vi "rotate_boat_overlays.vi"(8 "Overlay References In":T3, 9 "Rudder Setpoint":T1 min=-0.95 max=0.95 scale=1.0..-1.0, 10 "Sail Setpoints":T2 {"MainSailSuggestion" min=0.0 max=1.0; "JibSailSuggestion" min=0.0 max=1.0}, 11 "Heading":dbl) -> (1 "Rotated Boat Icon Bitmap Out":u32[][](array[colorbox]), 3 "Boat Icon Out":T4(plugin-control))   [LabVIEW 2013]
doc: "Rotates icon images of the boat and sails and overlays them on each other to create a representation of the current state of the robot. Also converts the output image to a bitmap for easy overlay on the mission map.\n\norigininally by Jason Curtis\nAdapted 4/5/2014 by Mac-I Crowell"
uses:
  TypeDef/boat_overlay_references.ctl
  <vilib>/vision/Image Controls.llb/IMAQ Image.ctl
  cRIO_Code/Data/TypeDefs/Sail Set Suggestions.ctl
  cRIO_Code/Data/TypeDefs/Rudder Set Suggestions.ctl
  <vilib>/vision/NI_Vision_Development_Module.lvlib
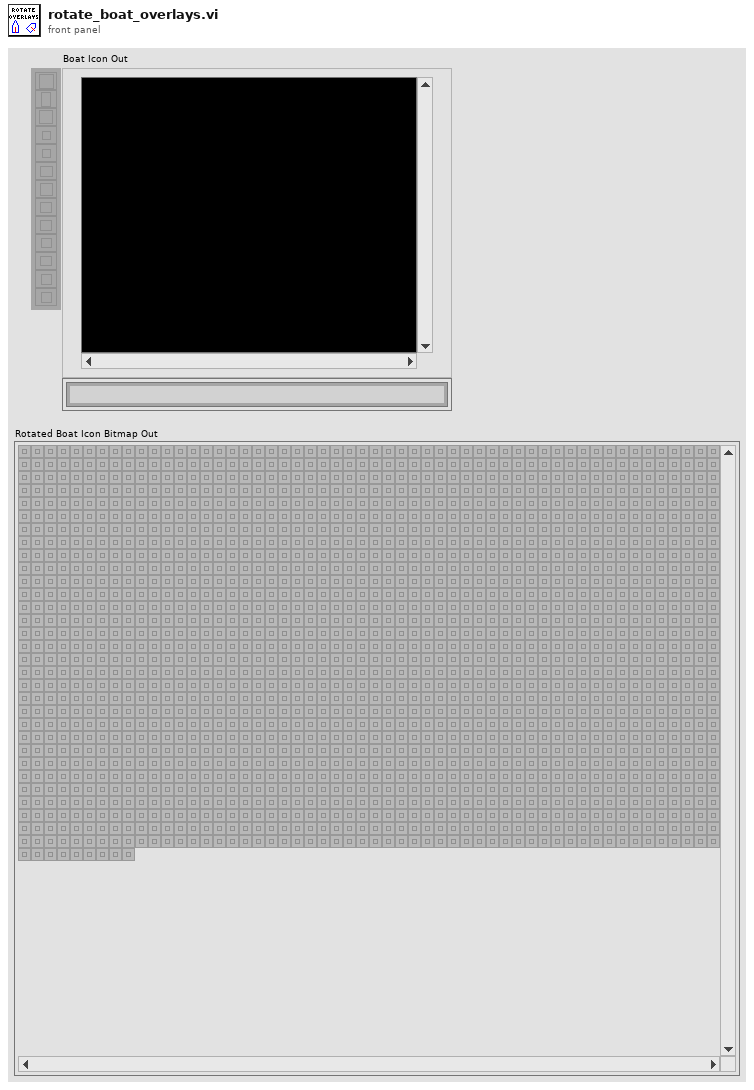
[diagram p1: front panel]
types:
  T1 = typedef "Rudder Set Suggestions.ctl" = dbl
  T2 = typedef "Sail Set Suggestions.ctl" = cluster{"MainSailSuggestion":dbl, "JibSailSuggestion":dbl}
  T3 = typedef "boat_overlay_references.ctl" = cluster{"Boat Icon, Unrotated":T4, "Boat Icon, Rotated":T4, "Mainsail Icon, Unrotated":T4, "Mainsail Icon, Rotated":T4, "Jib Icon, Rotated":T4, "Jib Icon, Unrotated":T4, "Rudder Icon, Rotated":T4, "Rudder Icon, Unrotated":T4}
  T4 = typedef "IMAQ Image.ctl" = refnum<image>
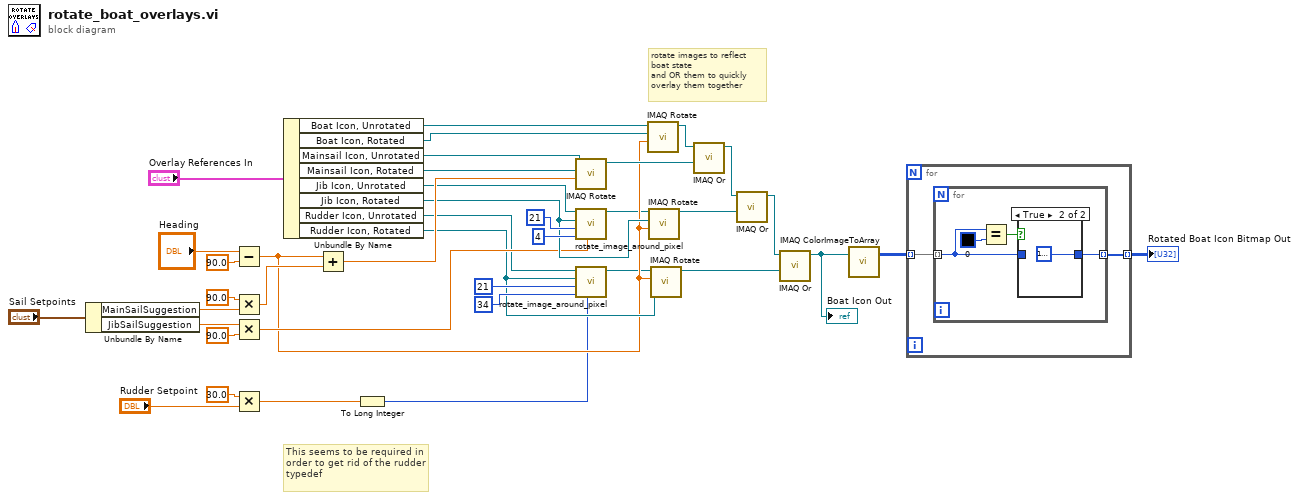
[diagram p0: block diagram]
diagram:
  # "This seems to be required in order to get rid of the rudder typedef"
  # "rotate images to reflect\nboat state\nand OR them to quickly \noverlay them together"
  n1 = Unbundle By Name("Sail Setpoints") -> ("MainSailSuggestion"=w24:dbl, "JibSailSuggestion"=w21:dbl)
  n2 = Subtract(x="Heading", y=90.0) -> (x-y=w8:dbl)
  n3 = Multiply(x=90.0 ("y"), y=w24) -> (x*y=w29:dbl)
  n4 = Multiply(x=w21, y=90.0) -> (x*y=w10:dbl)
  n5 = Multiply(x=30.0 ("y"), y="Rudder Setpoint") -> (x*y=w16:T1)
  n6 = Unbundle By Name("Overlay References In") -> ("Boat Icon, Unrotated"=w39:T4, "Boat Icon, Rotated"=w38:T4, "Mainsail Icon, Unrotated"=w36:T4, "Mainsail Icon, Rotated"=w37:T4, "Jib Icon, Unrotated"=w3:T4, "Jib Icon, Rotated"=w11:T4, "Rudder Icon, Unrotated"=w6:T4, "Rudder Icon, Rotated"=w9:T4)
  n7 = Add(x=w8, y=w29) -> (x+y=w30:dbl)
  n8 = To Long Integer(number=w16) -> (32bit integer=w7:i32)
  n9 = call "IMAQ Rotate"("Angle (degrees)"=w30, "Image Dst"=w37, "Image Src"=w36) -> ("Image Dst Out"=w34:T4)  [unwired: 7 in, 1 out]
  n10 = call "rotate_image_around_pixel.vi"("Angle (degrees)"=w10, "Y Pixel"=4, "X Pixel"=21, "Image Dst"=w11, "Image Src"=w3) -> ("Image Dst Out"=w2:T4)  [unwired: 6 in]
  n11 = call "rotate_image_around_pixel.vi"("Angle (degrees)"=w7, "Y Pixel"=34, "X Pixel"=21, "Image Dst"=w9, "Image Src"=w6) -> ("Image Dst Out"=w5:T4)  [unwired: 6 in]
  n12 = call "IMAQ Rotate"("Angle (degrees)"=w8, "Image Dst"=w38, "Image Src"=w39) -> ("Image Dst Out"=w33:T4)  [unwired: 7 in, 1 out]
  n13 = call "IMAQ Rotate"("Angle (degrees)"=w8, "Image Dst"=w11, "Image Src"=w2) -> ("Image Dst Out"=w1:T4)  [unwired: 7 in, 1 out]
  n14 = call "IMAQ Rotate"("Angle (degrees)"=w8, "Image Dst"=w9, "Image Src"=w5) -> ("Image Dst Out"=w4:T4)  [unwired: 7 in, 1 out]
  n15 = call "IMAQ Or"("Image Src B"=w34, "Image Src A"=w33) -> ("Image Dst Out"=w20:T4)  [unwired: 8 in, 1 out]
  n16 = call "IMAQ Or"("Image Src B"=w1, "Image Src A"=w20) -> ("Image Dst Out"=w19:T4)  [unwired: 8 in, 1 out]
  n17 = call "IMAQ Or"("Image Src B"=w4, "Image Src A"=w19) -> ("Image Dst Out"=w18:T4)  [unwired: 8 in, 1 out]
  "Boat Icon Out" <- w18
  n18 = call "IMAQ ColorImageToArray"("Image"=w18) -> ("Image Pixels (U32)"=w31:u32[][])  [unwired: 2 in, 3 out]
  n19 = for {
    tunnel: w31 -> [w41] mode=indexing
    tunnel: [w40] -> w32 mode=indexing
    n20 = for {
      tunnel: w41 -> [w43] mode=indexing
      tunnel: [w44] -> w40 mode=indexing
      n21 = Equal?(x=w43, y=u32 0) -> (x = y?=w45:bool)
      n22 = case shown="True" w45 {
        tunnel: [w46 u32 16777216] -> w44
        tunnel: w43 -> [w46 _]
        frame False {
        }
        frame True {
        }
      }
    }
  }
  "Rotated Boat Icon Bitmap Out" <- w32
